vi "gfitsio-get-image-size.vi"(8 "error in (no error)":errorcluster, 11 "gfits refnum":T1) -> (0 "error out":errorcluster, 1 "naxes":i32[](array[numeric]), 2 "naxis":i32, 3 "dup gfits refnum":T1)   [LabVIEW 2024, in "gfitsio.lvlib"]
doc: "Get the number of dimensions and the size,in elements, of each dimension in the current HDU. Returns an error if the current HDU is not an image."
uses:
  gfitsio.lvlib
  gfitsio-refnum.ctl
  gfitsio.dll
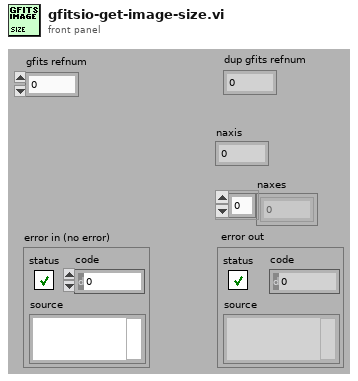
[diagram p1: front panel]
types:
  T1 = typedef "gfitsio.lvlib/gfitsio-refnum.ctl" = u64
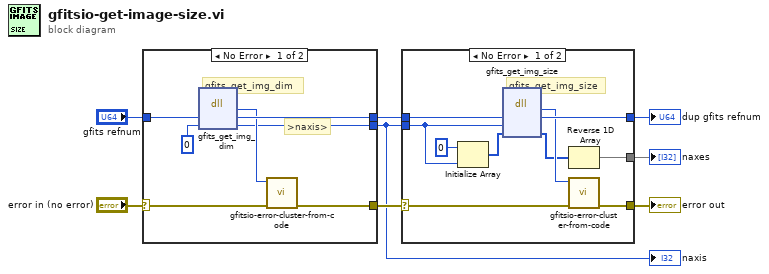
[diagram p0: block diagram]
diagram:
  n1 = case shown="No Error" "error in (no error)" {
    selector: "error in (no error)" -> [w13 w16]
    tunnel: "gfits refnum" -> [w12 w17]
    tunnel: [w10 _] -> w1
    tunnel: [w15 w17] -> w2
    tunnel: [w14 w16] -> w3
    frame No Error {
      # "gfits_get_img_dim"
      # ">naxis>"
      n2 = dll-call lib="C:/Development/rimas/RIMAS/gfitsio/gfitsio.dll" fn="gfits_get_img_dim"("handle"=w12, "naxis"=0) -> ("return type"=w11:i32, "handle"=w15:T1, "naxis"=w10:i32)  [unwired: 3 in, 2 out]
      n3 = call "gfitsio-error-cluster-from-code.vi"("error in (no error)"=w13, "error code"=w11) -> ("error out"=w14:errorcluster)  [unwired: 9 out]
    }
    frame Error {
    }
  }
  "naxis" <- w1
  n4 = case shown="No Error" w3 {
    selector: w3 -> [w18 w28]
    tunnel: w2 -> [w19 w29]
    tunnel: [w21 _] -> w6
    tunnel: [w26 w29] -> w8
    tunnel: [w24 w28] -> w7
    tunnel: w1 -> [w20 _]
    frame No Error {
      # "gfits_get_img_size"
      n5 = Initialize Array(0, w20) -> (w23:i32[])
      n6 = dll-call lib="C:/Development/rimas/RIMAS/gfitsio/gfitsio.dll" fn="gfits_get_img_size"("handle"=w19, "maxdim"=w20, "naxes"=w23) -> ("return type"=w25:i32, "handle"=w26:T1, "naxes"=w22:i32[])  [unwired: 4 in, 2 out]
      n7 = Reverse 1D Array(array=w22) -> (reversed array=w21:i32[])
      n8 = call "gfitsio-error-cluster-from-code.vi"("error in (no error)"=w18, "error code"=w25) -> ("error out"=w24:errorcluster)  [unwired: 9 out]
    }
    frame Error {
    }
  }
  "dup gfits refnum" <- w8
  "error out" <- w7
  "naxes" <- w6
